vi "Stop Module.vi"(8 "error in (no error)":errorcluster, 9 "Wait for Module to stop? (F)":bool, 10 "Origin":string, 11 "Module ID":i32=-1) -> (0 "error out":errorcluster)   [LabVIEW 2020, in "GenNet-Server.lvlib"]
doc: "Send the Stop request to the Module's Main.vi. If <b>Wait for Module to stop?</b> is TRUE, then this VI will not complete execution until the Module Main VI has stopped running.\n\n<b>Note:</b> If the cloneable module is running as singleton, then the 'Wait for Module to stop?' input is ignored... this VI will <b>always</b> wait until a cloneable Main VI running as singleton has stopped running.\n\n<b>Note:</b> This VI was modified by the <b>Validate DQMH Module</b> tool to upgrade it to the DQMH 5.1 approach to poll the execution state of a cloneable module running as singleton to know when the module has gone idle.\n\n<b>Note:</b> This VI was modified by the <b>Validate DQMH Module</b> tool to upgrade it to the DQMH 5.0 approach to destroying cloneable module event references.\n\n<b>Note:</b> This VI was modified by the <b>Validate DQMH Module</b> tool to remove the Status Updated.vi subVI call.\n\n____\nHAMPEL SOFTWARE ENGINEERING v3.8.0 (2023-12-18 14:41)"
uses:
  GenNet-Server.lvlib
  Stop Argument--cluster.ctl
  Module Running State--enum.ctl
  Main.vi
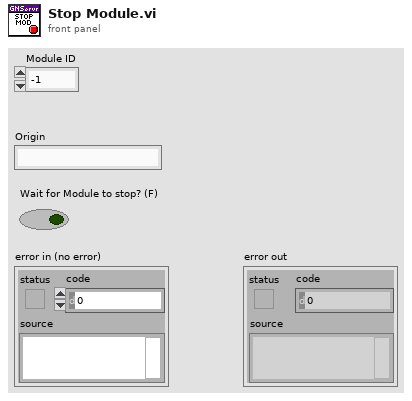
[diagram p1: front panel]
types:
  T1 = typedef "GenNet-Server.lvlib/Module Running State--enum.ctl" = enum16{"Not Running", "Running as Cloneable", "Running as Singleton"}
  T2 = typedef "GenNet-Server.lvlib/Stop Argument--cluster.ctl" = cluster{"Origin":string, "Module ID":i32, "Exit via Stop Module Req?":bool, "Wait for Module to stop?":bool}
  T3 = typedef "GenNet-Server.lvlib/Request Events--cluster.ctl" = cluster{"Stop Module":refnum<user-event>, "Show Panel":refnum<user-event>, "Hide Panel":refnum<user-event>, "Show Diagram":refnum<user-event>, "Get Module Execution Status":refnum<user-event>, "Forward Generic Broadcasts to Network":refnum<user-event>}
  T4 = enum32{"Bad", "Idle", "Run top level", "Running"}
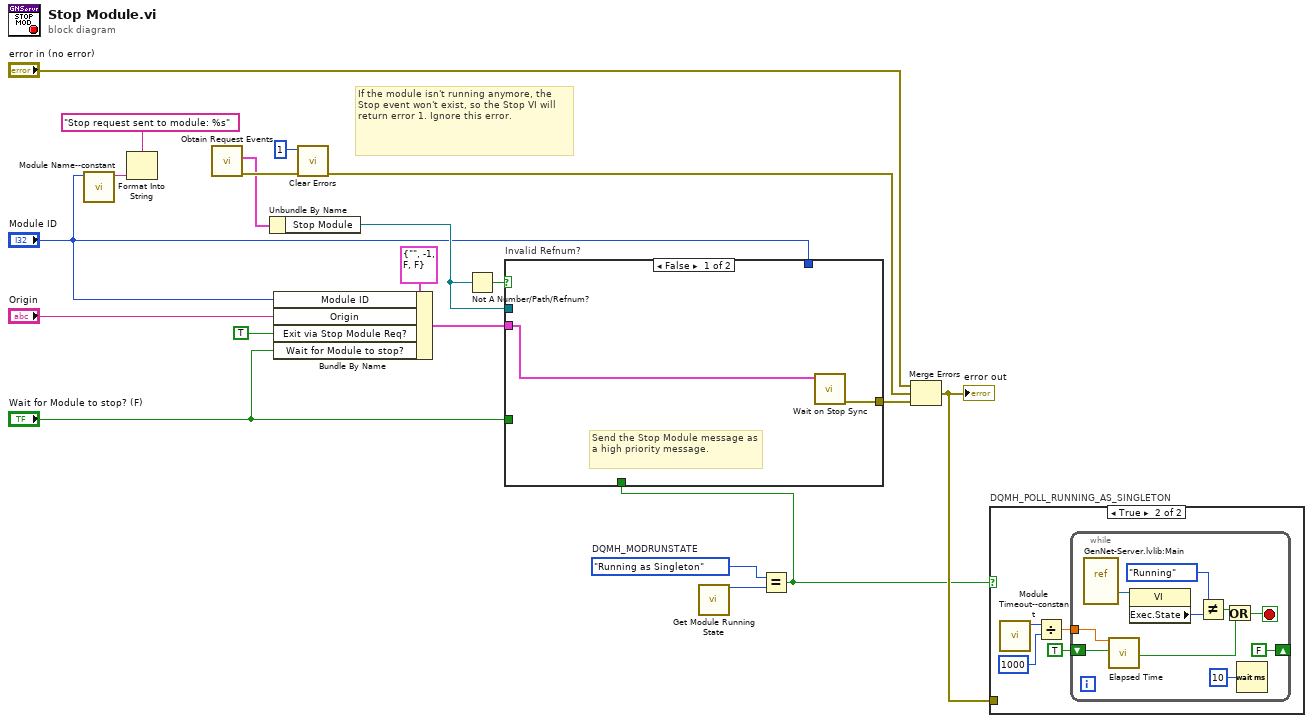
[diagram p0: block diagram]
diagram:
  w2 = Module_Running_State--enum."Running as Singleton"  # DQMH_MODRUNSTATE
  # "If the module isn't running anymore, the Stop event won't exist, so the Stop VI will return error 1. Ignore this error."
  n1 = call "Module Name--constant.vi"("Module ID"="Module ID") -> ("Module Name"=w18:string)  [unwired: 10 in]
  n2 = Format Into String(format string="Stop request sent to module: %s", w18) -> ()  [unwired: 2 in, 2 out]
  n3 = call "Obtain Request Events.vi"() -> ("error out"=w11:errorcluster, "GenNet-Server Request Events"=w9:T3)  [unwired: 10 in]
  n4 = Unbundle By Name(w9) -> ("Stop Module"=w13:refnum<user-event>)
  n5 = Bundle By Name(cluster=T2 {"Origin"="", "Module ID"=-1, "Exit via Stop Module Req?"=FALSE, "Wait for Module to stop?"=FALSE} ("event data"), "Module ID"="Module ID", "Origin"="Origin", "Exit via Stop Module Req?"=TRUE, "Wait for Module to stop?"="Wait for Module to stop? (F)") -> (w12:T2)
  n6 = call <vilib>:"Clear Errors.vi"("error in (no error)"=w11, "specific error code to clear (0: all)"=1) -> ("error out"=w8:errorcluster)  [unwired: 4 in, 1 out]
  n7 = Not A Number/Path/Refnum?(number/path/refnum=w13) -> (NaN/Path/Refnum?=w14:bool)
  n8 = call "Get Module Running State.vi"() -> ("Module Running State"=w1:T1)  [unwired: 11 in]
  n9 = Equal?(x=w2, y=w1) -> (x = y?=w3:bool)
  n10 = case "Invalid Refnum?" shown="False" w14 {
    tunnel: [w21 _] -> w7
    tunnel: w12 -> [w22 _]
    tunnel: w13 -> [_ _]
    tunnel: "Module ID" -> [_ _]
    tunnel: "Wait for Module to stop? (F)" -> [_ _]
    tunnel: w3 -> [_ _]
    frame False {
      # "Send the Stop Module message as a high priority message."
      n11 = call "Wait on Stop Sync.vi"("Stop Argument"=w22) -> ("error out"=w21:errorcluster)  [unwired: 10 in]
    }
    frame True {
      # "Module is exiting. No need to send the standard \"not running\" error that is sent in other request VIs."
    }
  }
  n12 = Merge Errors("error in (no error)", w8, w7) -> (w15:errorcluster)
  "error out" <- w15
  n13 = case "DQMH_POLL_RUNNING_AS_SINGLETON" shown="True" w3 {
    tunnel: w15 -> [_ _]
    frame False {
    }
    frame True {
      n14 = call "Module Timeout--constant.vi"() -> ("Module Timeout"=w23:i32)  [unwired: 11 in]
      n15 = Divide(x=w23, y=1000) -> (x/y=w25:dbl)
      n16 = while {
        tunnel: w25 -> [w30]
        shift-right: [FALSE] -> _
        shift-left: TRUE -> [w31]
        stop <- w33 stop-if-true
        n17 = vi-ref "GenNet-Server.lvlib:Main.vi"() -> (w28:refnum<vi>)
        n18 = call "Elapsed Time"("Time Target (s)"=w30, "Reset"=w31) -> ("Time has Elapsed"=w29:bool)  [unwired: 10 in, 7 out]
        n19 = property class="VI"(reference=w28) -> ("Exec.State"=w36:T4)  [unwired: 1 in, 2 out]
        n20 = Not Equal?(x=T4."Running", y=w36) -> (x != y?=w34:bool)
        n21 = Or(x=w34, y=w29) -> (x .or. y?=w33:bool)
        n22 = Wait (ms)(milliseconds to wait=u32 10) -> ()  [unwired: 1 out]
      }
    }
  }
